vi "Fiducial Autofocus.vi"(8 "Image":T1(plugin-control), 11 "Gantry In":refnum<k24>) -> (3 "Gantry Out":refnum<k24>)   [LabVIEW 2021, in "Test VIs.lvclass"]
uses:
  Test VIs/Test VIs.lvclass
  Classes/Controller/Motion/A3200/A3200.lvclass
  Classes/Controller/Controller.lvclass
  C:/Program Files (x86)/Aerotech/A3200/LabVIEW/2010/Bin/Aerotech.A3200.dll
  Program Files (x86)/Aerotech/A3200/LabVIEW/2010/Bin/Aerotech.A3200.dll
panel:
  out "Current position":dbl[](array[numeric])
  in  "X, Y pixel stride":dbl[](array[numeric])=[1520.0, 2160.0]
  in  "Loop count":dbl=1.0
  out "Current position 2":dbl[](array[numeric])
  in  "X, Y pixel stride 2":dbl[](array[numeric])=[1520.0, 2160.0]
  in  "Loop count 2":dbl=1.0
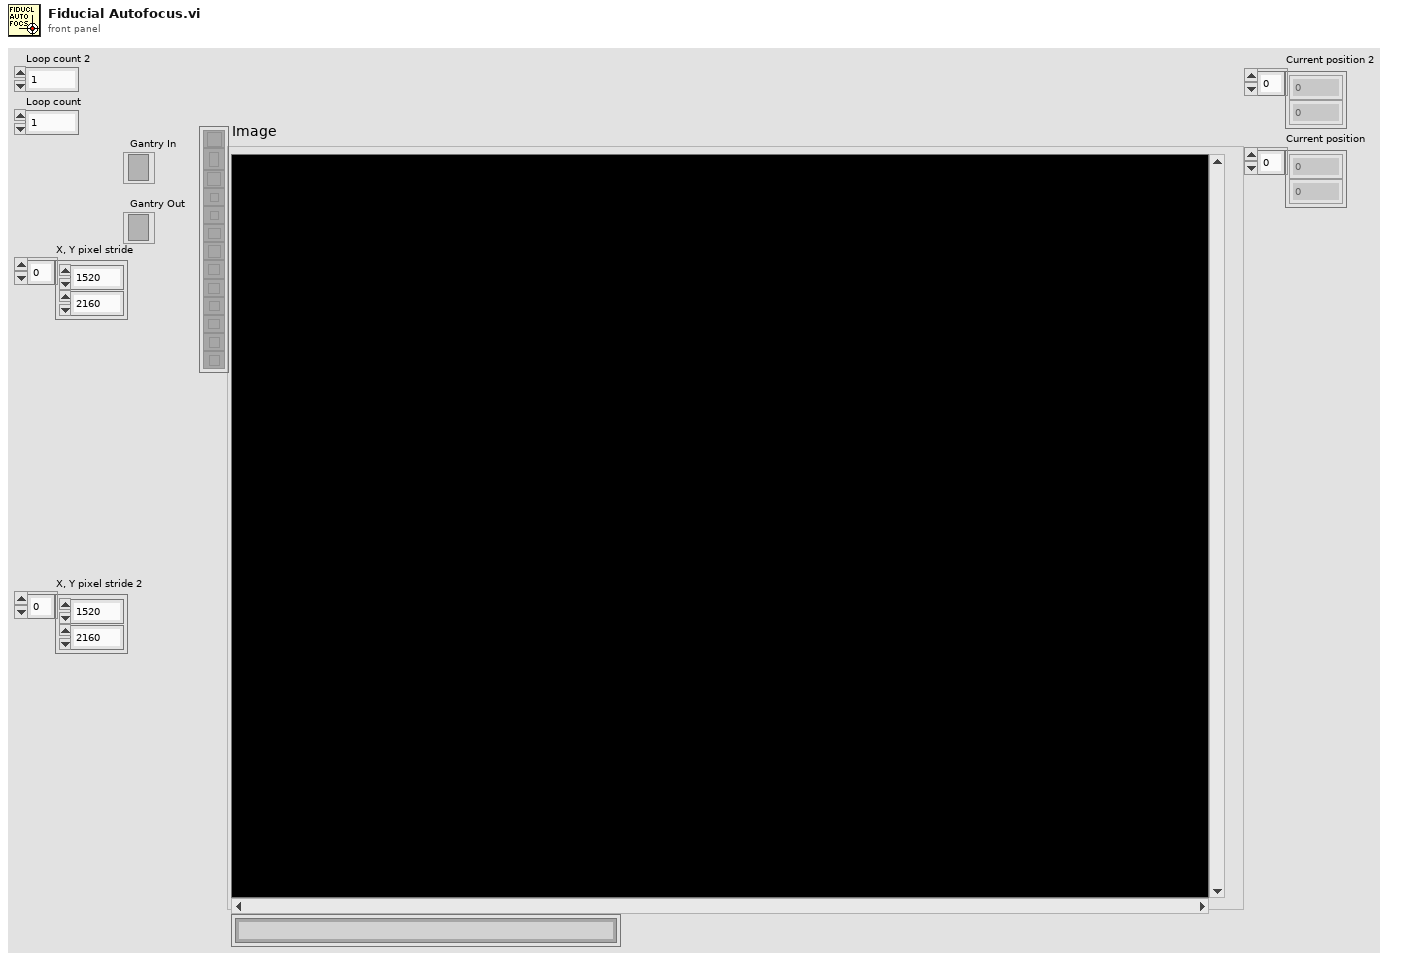
[diagram p1: front panel]
types:
  T1 = typedef "IMAQ Image.ctl" = refnum<image>
  T2 = typedef "Controller.lvclass/Controllers.ctl" = cluster{"I-O.lvclass":refnum<class "I-O.lvclass">, "Gantry":refnum<k24>, "Dispenser":refnum<visa-resource-name>}
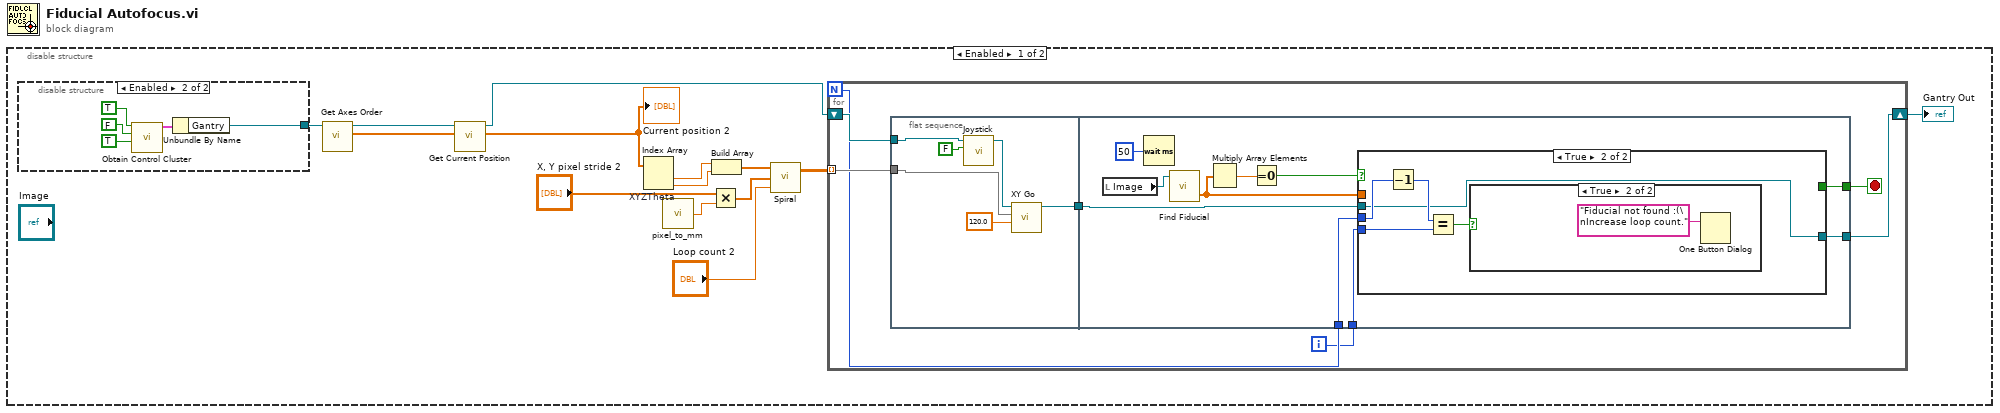
[diagram p0: block diagram]
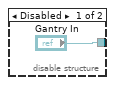
[diagram p2: hidden frame]
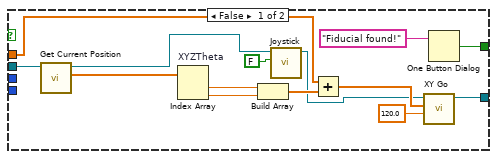
[diagram p3: hidden frame]
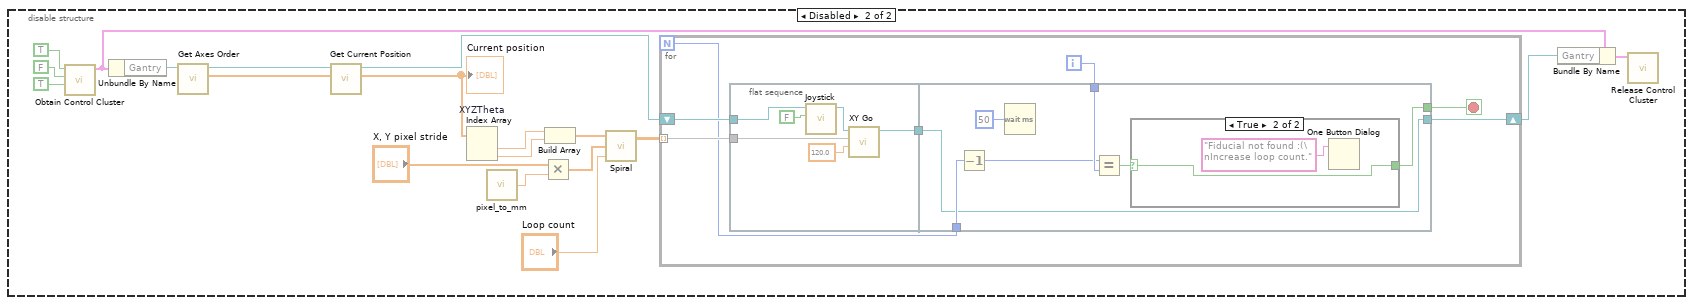
[diagram p5: hidden frame]
diagram:
  n1 = disable-structure shown="Enabled" {
    frame Enabled {
      n2 = disable-structure shown="Enabled" {
        disable-tunnel: ["Gantry In" w16] -> w3
        frame Disabled {
        }
        frame Enabled {
          n3 = call "Obtain Control Cluster.vi"("I/O"=TRUE ("Dispense"), "Dispense"=FALSE, "Motion"=TRUE ("I/O")) -> ("Control Out"=w17:T2)  [unwired: 7 in, 1 out]
          n4 = Unbundle By Name(w17) -> ("Gantry"=w16:refnum<k24>)
        }
      }
      n5 = call "Get Axes Order.vi"("Gantry In"=w3) -> ("Axes Order"=w2:dbl[], "Gantry Out"=w1:refnum<k24>)  [unwired: 8 in, 1 out]
      n6 = call "Get Current Position.vi"(10:w2, "Gantry In"=w1) -> ("XYZTheta Out"=w6:dbl[], "Gantry Out"=w4:refnum<k24>)  [unwired: 7 in, 1 out]
      "Current position 2" <- w6
      n7 = Index Array "XYZTheta"(array=w6) -> (element #1=w13:dbl, element #2=w12:dbl)  [unwired: 2 in]
      n8 = call "pixel_to_mm.vi"() -> ("mm/pixel"=w11:dbl)  [unwired: 2 in]
      n9 = Multiply(x="X, Y pixel stride 2", y=w11) -> (x*y=w8:dbl[])
      n10 = Build Array(w13, w12) -> (w7:dbl[])
      n11 = call "Spiral.vi"("Loop count"="Loop count 2", "X, Y stride (mm)"=w8, "XY center (mm)"=w7) -> ("Spiral coordinates"=w5:dbl[][])  [unwired: 1 in]
      n12 = for {
        N -> [w23]
        tunnel: w5 -> [w27] mode=indexing
        shift-right: [w25] -> w14
        shift-left: w4 -> [w26]
        i -> [w22]
        stop <- w24 stop-if-true
        n13 = flat-sequence {
          tunnel: [w28] -> w21
          tunnel: w26 -> [w30]
          tunnel: w27 -> [w29]
          tunnel: [w40] -> w25
          tunnel: [w42] -> w24
          tunnel: w23 -> [w39]
          tunnel: w22 -> [w38]
          tunnel: w21 -> [w37]
          frame #0 {
            n14 = call "Joystick.vi"("Joystick"=FALSE, "Gantry In"=w30) -> ("Gantry Out"=w33:refnum<k24>)  [unwired: 8 in, 1 out]
            n15 = call "XY Go.vi"("Speed"=120.0, "XY In"=w29, "Gantry In"=w33) -> ("Gantry Out"=w28:refnum<k24>)  [unwired: 6 in, 2 out]
          }
          frame #1 {
            n16 = local read "Image"() -> (w43:T1)
            n17 = Wait (ms)(milliseconds to wait=u32 50) -> ()  [unwired: 1 out]
            n18 = call "Find Fiducial.vi"("Image"=w43) -> ("Move by (mm)"=w41:dbl[])  [unwired: 3 in]
            n19 = Multiply Array Elements(1:w41) -> (0:w35:dbl)
            n20 = Equal To 0?(x=w35) -> (x = 0?=w34:bool)
            n21 = case shown="True" w34 {
              tunnel: [w47 _] -> w42
              tunnel: w41 -> [w46 _]
              tunnel: [w45 w58] -> w40
              tunnel: w39 -> [_ w60]
              tunnel: w38 -> [_ w59]
              tunnel: w37 -> [w44 w58]
              frame False {
                n22 = call "Get Current Position.vi"("Gantry In"=w44) -> ("XYZTheta Out"=w52:dbl[], "Gantry Out"=w57:refnum<k24>)  [unwired: 8 in, 1 out]
                n23 = Index Array "XYZTheta"(array=w52) -> (element #1=w53:dbl, element #2=w54:dbl)  [unwired: 2 in]
                n24 = Build Array(w53, w54) -> (w55:dbl[])
                n25 = call "Joystick.vi"("Joystick"=FALSE, "Gantry In"=w57) -> ("Gantry Out"=w51:refnum<k24>)  [unwired: 8 in, 1 out]
                n26 = Add(x=w46, y=w55) -> (x+y=w56:dbl[])
                n27 = call "XY Go.vi"("Speed"=120.0, "XY In"=w56, "Gantry In"=w51) -> ("Gantry Out"=w45:refnum<k24>)  [unwired: 6 in, 2 out]
                n28 = One Button Dialog(message="Fiducial found!") -> (true=w47:bool)  [unwired: 1 in]
              }
              frame True {
                n29 = Decrement(x=w60) -> (x-1=w62:i32)
                n30 = Equal?(x=w62, y=w59) -> (x = y?=w61:bool)
                n31 = case shown="True" w61 {
                  frame False {
                  }
                  frame True {
                    n32 = One Button Dialog(message="Fiducial not found :(\nIncrease loop count.") -> ()  [unwired: 1 in, 1 out]
                  }
                }
              }
            }
          }
        }
      }
      "Gantry Out" <- w14
    }
    frame Disabled {
      n33 = call "Obtain Control Cluster.vi"("I/O"=TRUE ("Dispense"), "Dispense"=FALSE, "Motion"=TRUE ("I/O")) -> ("Control Out"=w64:T2)  [unwired: 7 in, 1 out]
      n34 = Unbundle By Name(w64) -> ("Gantry"=w71:refnum<k24>)
      n35 = call "Get Axes Order.vi"("Gantry In"=w71) -> ("Axes Order"=w70:dbl[], "Gantry Out"=w69:refnum<k24>)  [unwired: 8 in, 1 out]
      n36 = call "Get Current Position.vi"(10:w70, "Gantry In"=w69) -> ("XYZTheta Out"=w75:dbl[], "Gantry Out"=w68:refnum<k24>)  [unwired: 7 in, 1 out]
      "Current position" <- w75
      n37 = Index Array "XYZTheta"(array=w75) -> (element #1=w82:dbl, element #2=w81:dbl)  [unwired: 2 in]
      n38 = call "pixel_to_mm.vi"() -> ("mm/pixel"=w80:dbl)  [unwired: 2 in]
      n39 = Multiply(x="X, Y pixel stride", y=w80) -> (x*y=w77:dbl[])
      n40 = Build Array(w82, w81) -> (w76:dbl[])
      n41 = call "Spiral.vi"("Loop count"="Loop count", "X, Y stride (mm)"=w77, "XY center (mm)"=w76) -> ("Spiral coordinates"=w67:dbl[][])  [unwired: 1 in]
      n42 = for {
        N -> [w85]
        tunnel: w67 -> [w89] mode=indexing
        shift-right: [w87] -> w65
        shift-left: w68 -> [w88]
        i -> [w84]
        stop <- w86 stop-if-true
        n43 = flat-sequence {
          tunnel: [w90] -> w83
          tunnel: w88 -> [w92]
          tunnel: w89 -> [w91]
          tunnel: [w100] -> w87
          tunnel: [w96] -> w86
          tunnel: w85 -> [w102]
          tunnel: w84 -> [w101]
          tunnel: w83 -> [w100]
          frame #0 {
            n44 = call "Joystick.vi"("Joystick"=FALSE, "Gantry In"=w92) -> ("Gantry Out"=w95:refnum<k24>)  [unwired: 8 in, 1 out]
            n45 = call "XY Go.vi"("Speed"=120.0, "XY In"=w91, "Gantry In"=w95) -> ("Gantry Out"=w90:refnum<k24>)  [unwired: 6 in, 2 out]
          }
          frame #1 {
            n46 = Decrement(x=w102) -> (x-1=w98:i32)
            n47 = Wait (ms)(milliseconds to wait=u32 50) -> ()  [unwired: 1 out]
            n48 = Equal?(x=w98, y=w101) -> (x = y?=w97:bool)
            n49 = case shown="True" w97 {
              selector: w97 -> [w103 w104]
              tunnel: [w103 w104] -> w96
              frame False {
              }
              frame True {
                n50 = One Button Dialog(message="Fiducial not found :(\nIncrease loop count.") -> ()  [unwired: 1 in, 1 out]
              }
            }
          }
        }
      }
      n51 = Bundle By Name(cluster=w64, "Gantry"=w65) -> (w66:T2)
      n52 = call "Release Control Cluster.vi"("output cluster"=w66) -> ()  [unwired: 11 in]
    }
  }
